vi "PIMotorController.vi"(6 "SetPosition waittime (30)":u32=30, 9 "MotorConfig":T4={"Offset"={"Magnet Z"=0.0, "Magnet rotation"=0.0, "Camera"={"X"=0.0, "Y"=0.0}, "Piezo XY"={"X"=0.0, "Y"=0.0}, "Piezo Z"=0.0, "Coil XY"={"X"=0.0, "Y"=0.0}}, "Maximum pos"={"Magnet Z"=0.0, "Magnet rotation"=0.0, "Camera"={"X"=0.0, "Y"=0.0}, "Piezo XY"={"X"=0.0, "Y"=0.0}, "Piezo Z"=0.0, "Coil XY"={"X"=0.0, "Y"=0.0}}, "Min limited?"={"Magnet Z"=FALSE, "Magnet rotation"=FALSE, "Camera"={"X"=FALSE, "Y"=FALSE}, "Piezo XY"={"X"=FALSE, "Y"=FALSE}, "Piezo Z"=FALSE, "Coil XY"={"X"=FALSE, "Y"=FALSE}}, "Max limited?"={"Magnet Z"=FALSE, "Magnet rotation"=FALSE, "Camera"={"X"=FALSE, "Y"=FALSE}, "Piezo XY"={"X"=FALSE, "Y"=FALSE}, "Piezo Z"=FALSE, "Coil XY"={"X"=FALSE, "Y"=FALSE}}, "Has velocity support"={"Magnet Z"=TRUE, "Magnet rotation"=TRUE, "Camera"={"X"=FALSE, "Y"=FALSE}, "Piezo XY"={"X"=FALSE, "Y"=FALSE}, "Piezo Z"=FALSE, "Coil XY"={"X"=FALSE, "Y"=FALSE}}, "Default velocity"={"Magnet Z"=0.0, "Magnet rotation"=0.0, "Camera"={"X"=0.0, "Y"=0.0}, "Piezo XY"={"X"=0.0, "Y"=0.0}, "Piezo Z"=0.0, "Coil XY"={"X"=0.0, "Y"=0.0}}}, 10 "PI GCS Function\nReferences":T1, 11 "PI Axis config":T2={"Piezo X"={"System #"=0, "Axis ID"="", "Multiplier"=1.0}, "Piezo Y"={"System #"=0, "Axis ID"="", "Multiplier"=1.0}, "Piezo Z"={"System #"=0, "Axis ID"="", "Multiplier"=1.0}, "Magnet Z"={"System #"=0, "Axis ID"="", "Multiplier"=1.0}, "Magnet Rotation"={"System #"=0, "Axis ID"="", "Multiplier"=1.0}, "Objective X"={"System #"=0, "Axis ID"="", "Multiplier"=1.0}, "Objective Y"={"System #"=0, "Axis ID"="", "Multiplier"=1.0}}) -> ()   [LabVIEW 2011]
uses:
  Main/Motors/MotorConfigType.ctl
  Main/Motors/MotorPosType.ctl
  Main/Typedefs/XYf.ctl
  Main/Motors/MotorPosFlagsType.ctl
  PI_Axis_list.ctl
  PI_Axis.ctl
  GCS_Interface.ctl
  Main/Motors/MotorAxisEnum.ctl
  Main/Typedefs/CmdEnum_MotorIn.ctl
  Main/Typedefs/Cmd_MotorIn.ctl
  PIAxisInfoGlobal.vi
  Main/GlobalVariables.vi
panel:
  out "Magnet Z":dbl
  in  "Get z position":bool
  in  "Piezo pos wanted":dbl
  in  "Initialize":bool
  out "get pos time":dbl
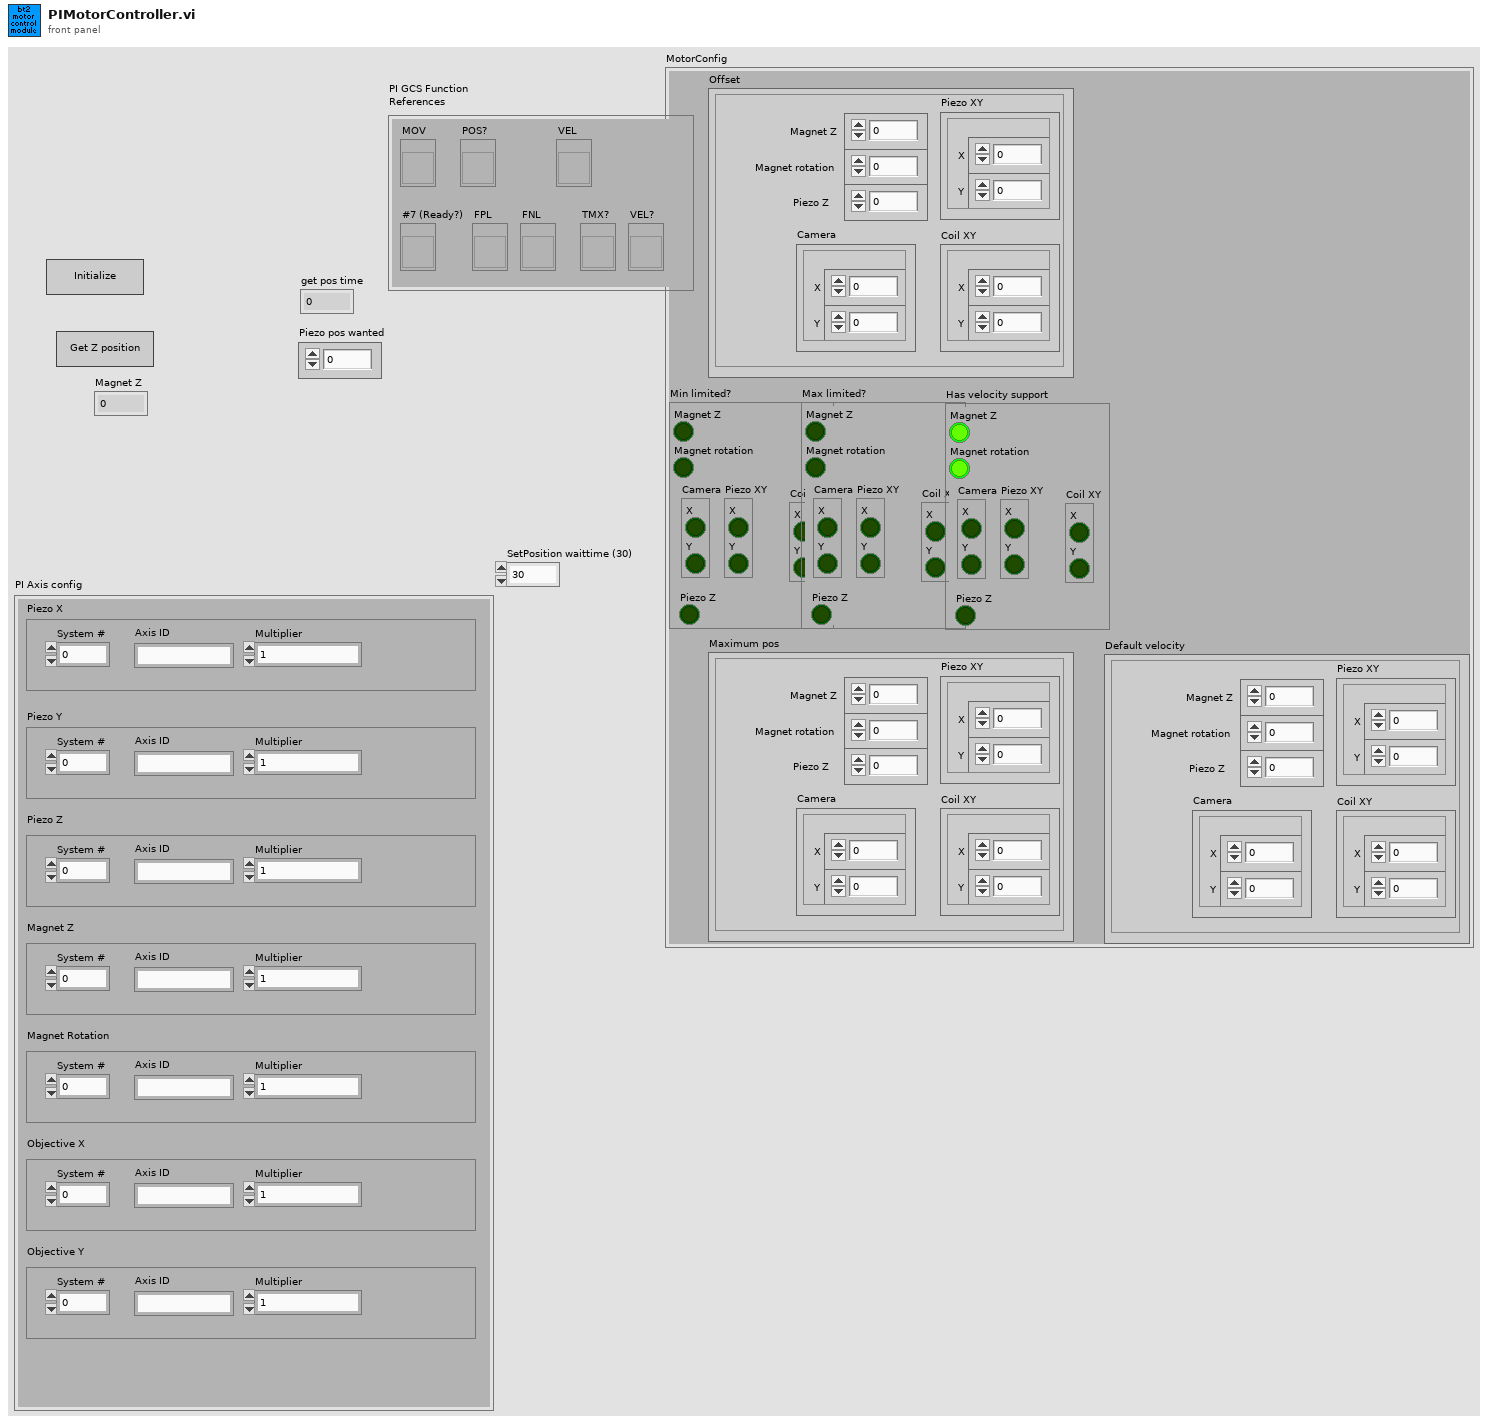
[diagram p1: front panel]
types:
  T1 = typedef "GCS_Interface.ctl" = cluster{"MOV":refnum<vi>, "VEL":refnum<vi>, "VEL?":refnum<vi>, "POS?":refnum<vi>, "TMX?":refnum<vi>, "#7 (Ready?)":refnum<vi>, "FPL":refnum<vi>, "FNL":refnum<vi>}
  T2 = typedef "PI_Axis_list.ctl" = cluster{"Piezo X":T3, "Piezo Y":T3, "Piezo Z":T3, "Magnet Z":T3, "Magnet Rotation":T3, "Objective X":T3, "Objective Y":T3}
  T3 = typedef "PI_Axis.ctl" = cluster{"System #":i32, "Axis ID":string, "Multiplier":dbl}
  T4 = typedef "MotorConfigType.ctl" = cluster{"Offset":T5, "Maximum pos":T5, "Min limited?":T7, "Max limited?":T7, "Has velocity support":T7, "Default velocity":T5}
  T5 = typedef "MotorPosType.ctl" = cluster{"Magnet Z":dbl, "Magnet rotation":dbl, "Camera":T6, "Piezo XY":T6, "Piezo Z":dbl, "Coil XY":T6}
  T6 = typedef "XYf.ctl" = cluster{"X":sgl, "Y":sgl}
  T7 = typedef "MotorPosFlagsType.ctl" = cluster{"Magnet Z":bool, "Magnet rotation":bool, "Camera":cluster{"X":bool, "Y":bool}, "Piezo XY":cluster{"X":bool, "Y":bool}, "Piezo Z":bool, "Coil XY":cluster{"X":bool, "Y":bool}}
  T8 = typedef "MotorAxisEnum.ctl" = enum16{"no axis", "magrot", "magpos", "px", "py", "pz", "camx", "camy"}
  T9 = typedef "QueueListType.ctl" = cluster{"Motor In":refnum<queue>, "User Interface Image View":refnum<queue>, "User Interface Camera Control":refnum<queue>, "User Interface Event Notifier":refnum<notifier>, "Initialized?":bool}
  T10 = typedef "CmdEnum_MotorIn.ctl" = enum32{"Init", "Close", "SetPosition", "UpdatePositions", "MoveToLimit"}
  T11 = typedef "Cmd_MotorIn.ctl" = cluster{"Command Type":T10, "Msg Data":variant}
  T12 = typedef "MotorStateType.ctl" = cluster{"Enabled?":bool, "Current Position":T5, "Update counter":i32}
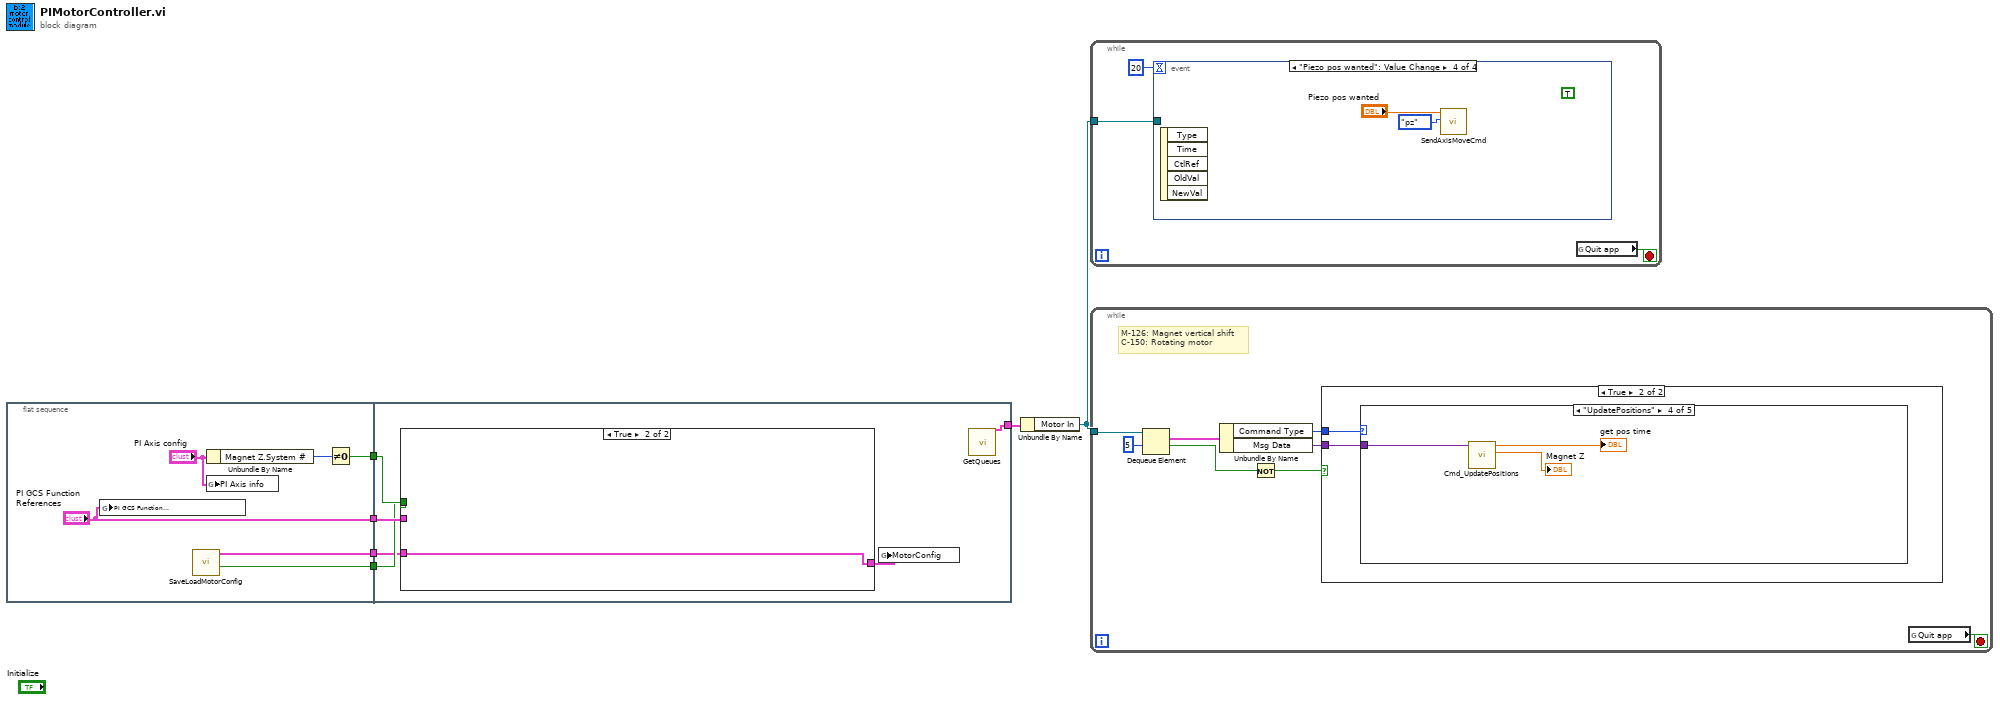
[diagram p0: block diagram]
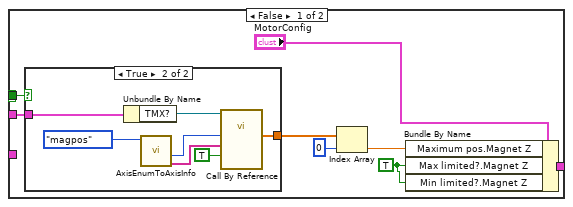
[diagram p2: hidden frame]
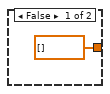
[diagram p3: hidden frame]
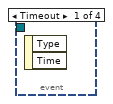
[diagram p4: hidden frame]
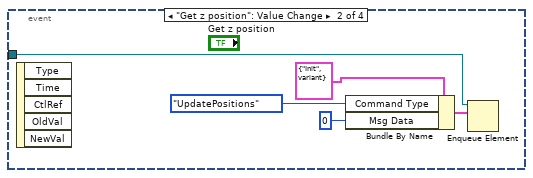
[diagram p5: hidden frame]
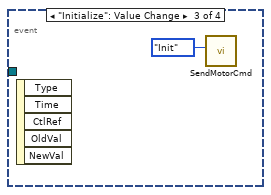
[diagram p6: hidden frame]
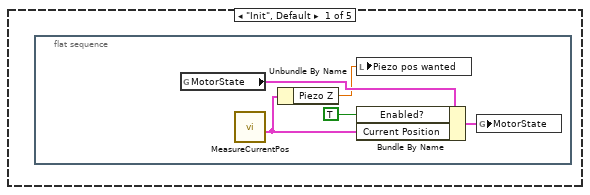
[diagram p8: hidden frame]
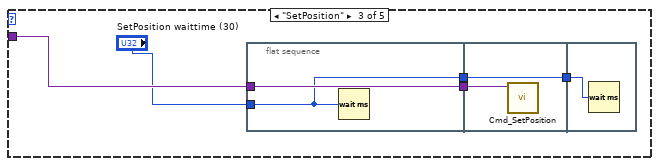
[diagram p10: hidden frame]
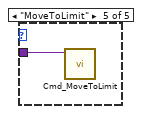
[diagram p11: hidden frame]
diagram:
  n1 = flat-sequence {
    tunnel: ["PI GCS Function\nReferences"] -> w5
    tunnel: [w9] -> w3
    tunnel: [w8] -> w2
    tunnel: [w7] -> w1
    tunnel: w5 -> [w18]
    tunnel: [w17] -> w4
    tunnel: w3 -> [w15]
    tunnel: w2 -> [w14]
    tunnel: w1 -> [w13]
    frame #0 {
      n2 = global write "PIAxisInfoGlobal.vi" "PI GCS Function\nReferences"("PI GCS Function\nReferences") -> ()
      n3 = call "SaveLoadMotorConfig.vi"() -> ("No error?"=w8:bool, "MotorConfig"=w7:T4)  [unwired: 9 in, 1 out]
      n4 = Unbundle By Name("PI Axis config") -> ("Magnet Z.System #"=w10:i32)
      n5 = global write "PIAxisInfoGlobal.vi" "PI Axis info"("PI Axis config") -> ()
      n6 = Not Equal To 0?(x=w10) -> (x != 0?=w9:bool)
    }
    frame #1 {
      n7 = case shown="True" w14 {
        tunnel: w18 -> [w26 _]
        tunnel: [w21 w35] -> w16
        tunnel: w15 -> [w20 _]
        tunnel: w13 -> [_ w35]
        frame False {
          w19 = TRUE ("Max limited?.Magnet Z")
          n8 = case shown="True" w20 {
            tunnel: w26 -> [_ w32]
            tunnel: [dbl[] [] ("Maximum travel limit") w28] -> w25
            frame False {
            }
            frame True {
              n9 = Unbundle By Name(w32) -> ("TMX?"=w33:refnum<vi>)
              n10 = call "AxisEnumToAxisInfo.vi"("Motor Axis"=MotorAxisEnum."magpos") -> ("Axis ID"=w30:string[], "System #"=w31:i32)  [unwired: 6 in, 3 out]
              n11 = call-by-ref "?"(reference=w33, "System no."=w31, "Axes to query"=w30, "Axis identifier?"=TRUE) -> ("Maximum travel limit"=w28:dbl[])  [unwired: 16 in, 3 out]
            }
          }
          n12 = Index Array(array=w25, index=0) -> (element=w22:dbl)
          n13 = Bundle By Name(cluster="MotorConfig", "Maximum pos.Magnet Z"=w22, "Max limited?.Magnet Z"=w19, "Min limited?.Magnet Z"=w19) -> (w21:T4)
        }
        frame True {
        }
      }
      n14 = global write "GlobalVariables.vi" "MotorConfig"(w16) -> ()
      n15 = call "GetQueues.vi"() -> ("Queue List"=w17:T9)  [unwired: 10 in, 1 out]
    }
  }
  n16 = Unbundle By Name(w4) -> ("Motor In"=w6:refnum<queue>)
  n17 = while {
    tunnel: w6 -> [w36]
    stop <- w38 stop-if-true
    n18 = event shown="[3] \"Piezo pos wanted\": Value Change" {
      selector: _ -> [_ _ _ _]
      dyn-events: _ -> [_ _ _ _]
      timeout: 20 -> [_ _ _ _]
      tunnel: w36 -> [_ w43 _ _]
      event Timeout {
        n19 = event-data() -> ()  [unwired: 1 in, 2 out]
      }
      event "Get z position": Value Change {
        n20 = event-data() -> ()  [unwired: 1 in, 5 out]
        n21 = Bundle By Name(cluster=T11 {"Command Type"=enum."Init", "Msg Data"=variant} ("element"), "Command Type"=CmdEnum_MotorIn."UpdatePositions", "Msg Data"=0 ("Update counter")) -> (w41:T11)
        n22 = Enqueue Element(queue=w43, element=w41) -> ()  [unwired: 2 in, 3 out]
      }
      event "Initialize": Value Change {
        n23 = event-data() -> ()  [unwired: 1 in, 5 out]
        n24 = call "SendMotorCmd.vi"("Command Type"=CmdEnum_MotorIn."Init") -> ()  [unwired: 11 in]
      }
      event "Piezo pos wanted": Value Change {
        (unwired) TRUE ("Piezo? (F)")
        n25 = event-data() -> ()  [unwired: 1 in, 5 out]
        n26 = call "SendAxisMoveCmd.vi"("axis"=MotorAxisEnum."pz", "Position"="Piezo pos wanted") -> ()  [unwired: 9 in, 1 out]
      }
    }
    n27 = global read "GlobalVariables.vi" "Quit app"() -> (w38:bool)
  }
  n28 = while {
    tunnel: w6 -> [w53]
    stop <- w54 stop-if-true
    # "M-126: Magnet vertical shift\nC-150: Rotating motor"
    n29 = Dequeue Element(queue=w53, timeout in ms (-1)=5) -> (element=w52:T11, timed out?=w48:bool)  [unwired: 1 in, 2 out]
    n30 = Unbundle By Name(w52) -> ("Command Type"=w51:T10, "Msg Data"=w50:variant)
    n31 = Not(x=w48) -> (.not. x?=w47:bool)
    n32 = case shown="True" w47 {
      tunnel: w51 -> [_ w56]
      tunnel: w50 -> [_ w55]
      frame False {
      }
      frame True {
        n33 = case shown="\"UpdatePositions\"" w56 {
          tunnel: w55 -> [_ _ w66 w73 w75]
          frame "Init", Default {
            n34 = flat-sequence {
              frame #0 {
                n35 = global read "GlobalVariables.vi" "MotorState"() -> (w61:T12)
                n36 = call "MeasureCurrentPos.vi"() -> ("Current Position"=w58:T5)  [unwired: 11 in]
                n37 = Unbundle By Name(w58) -> ("Piezo Z"=w57:dbl)
                n38 = local write "Piezo pos wanted"(w57) -> ()
                n39 = Bundle By Name(cluster=w61, "Enabled?"=TRUE, "Current Position"=w58) -> (w60:T12)
                n40 = global write "GlobalVariables.vi" "MotorState"(w60) -> ()
              }
            }
          }
          frame "Close" {
          }
          frame "SetPosition" {
            n41 = flat-sequence {
              tunnel: w66 -> [w68]
              tunnel: [w68] -> w65
              tunnel: "SetPosition waittime (30)" -> [w67]
              tunnel: [w67] -> w63
              tunnel: w65 -> [w70]
              tunnel: w63 -> [w69]
              tunnel: [w69] -> w62
              tunnel: w62 -> [w71]
              frame #0 {
                n42 = Wait (ms)(milliseconds to wait=w67) -> ()  [unwired: 1 out]
              }
              frame #1 {
                n43 = call "Cmd_SetPosition.vi"("Msg Data"=w70) -> ()  [unwired: 11 in]
              }
              frame #2 {
                n44 = Wait (ms)(milliseconds to wait=w71) -> ()  [unwired: 1 out]
              }
            }
          }
          frame "UpdatePositions" {
            n45 = call "Cmd_UpdatePositions.vi"("Msg Data"=w73) -> ("Magnet Z"=→"Magnet Z":dbl, "Numeric"=→"get pos time":dbl)  [unwired: 9 in]
          }
          frame "MoveToLimit" {
            n46 = call "Cmd_MoveToLimit.vi"("Msg Data"=w75) -> ()  [unwired: 11 in]
          }
        }
      }
    }
    n47 = global read "GlobalVariables.vi" "Quit app"() -> (w54:bool)
  }
